vi "databasehandle.vi"(7 "condition":string, 8 "error in (no error)":errorcluster caption="错误输入（无错误）", 9 "columns":string[](array[string]), 10 "password":string="123", 11 "table":string) -> (0 "error out":errorcluster caption="错误输出", 3 "data":string[][](array[string]))   [LabVIEW 2016, in "潮位站数据传输.lvlib"]
uses:
  access/access.lvclass
  database_class/database.lvclass/database.ctl
  database_class/database.lvclass
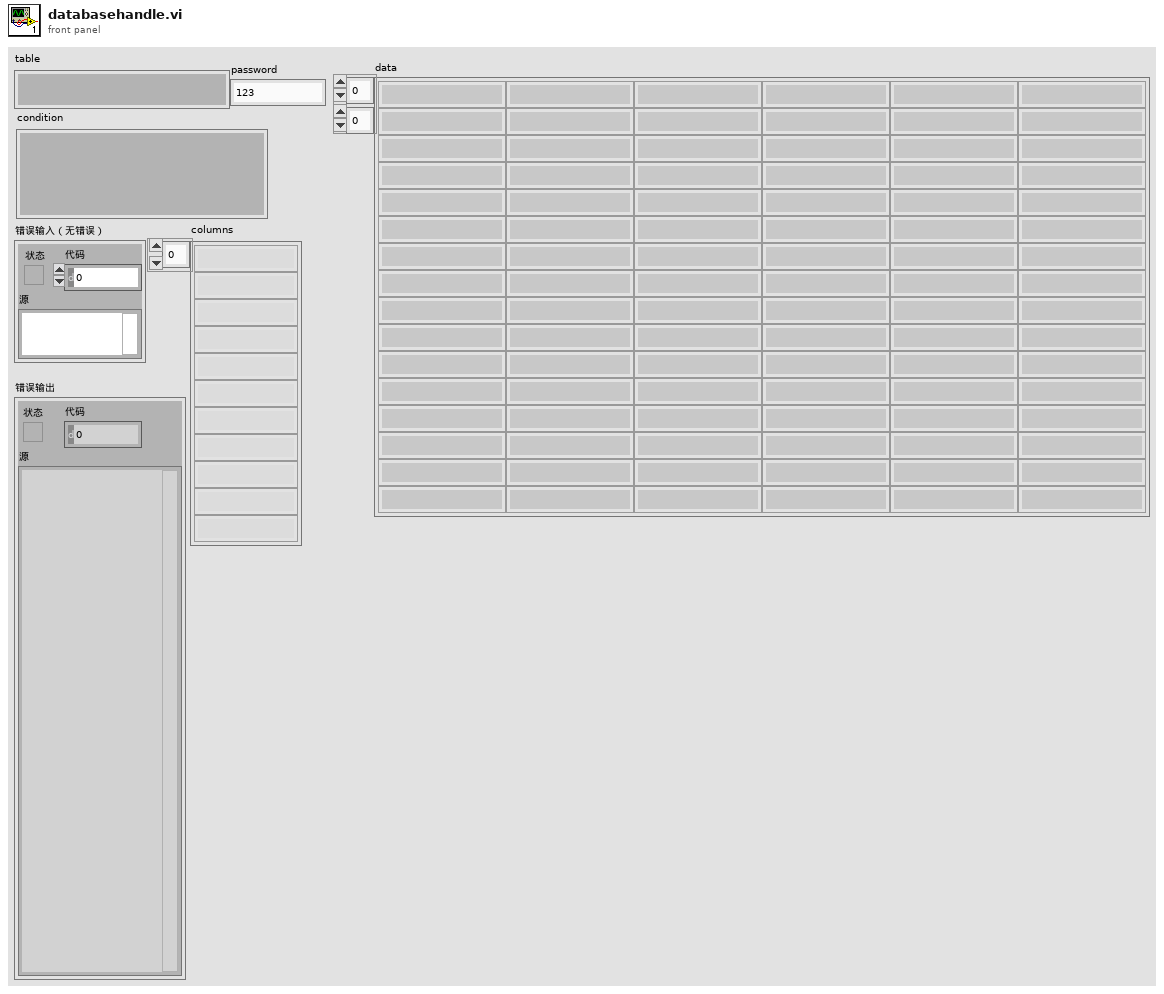
[diagram p1: front panel]
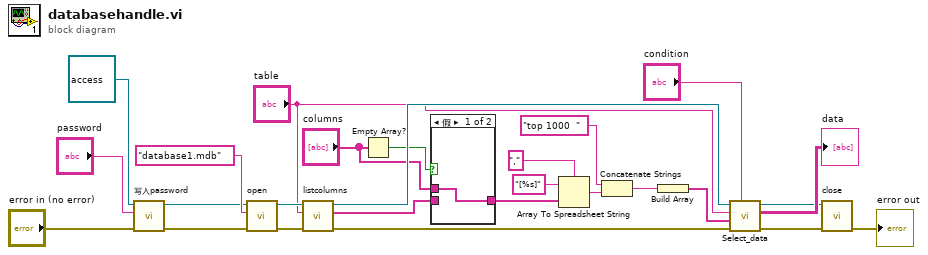
[diagram p0: block diagram]
diagram:
  n1 = call "写入password.vi"("error in (no error)"="error in (no error)", "password"="password", "database输入"=refnum<class "access.lvclass"> refnum ("access.lvclass")) -> ("error out"=w21:errorcluster, "database输出"=w23:refnum<class "access.lvclass">)  [unwired: 7 in]
  n2 = call-dynamic "open.vi"("error in (no error)"=w21, "database"="database1.mdb", "access 输入"=w23) -> ("error out"=w19:errorcluster, "access 输出"=w20:refnum<class "access.lvclass">)  [unwired: 7 in]
  n3 = call-dynamic "listcolumns.vi"("error in (no error)"=w19, "table"="table", "access 输入"=w20) -> ("error out"=w17:errorcluster, "columns"=w9:string[], "access 输出"=w18:refnum<class "access.lvclass">)  [unwired: 6 in]
  n4 = Empty Array?(array="columns") -> (empty?=w10:bool)
  n5 = case shown="假" w10 {
    tunnel: w9 -> [_ w28]
    tunnel: [w27 w28] -> w2
    tunnel: "columns" -> [w27 _]
    frame False {
    }
    frame True {
    }
  }
  n6 = Array To Spreadsheet String(delimiter (Tab)="," ("分隔符(Tab)"), array=w2, 3:"[%s]" ("格式字符串")) -> (spreadsheet string=w4:string)
  n7 = Concatenate Strings("top 1000  " ("字符串"), w4) -> (w3:string)
  n8 = Build Array(w3) -> (w1:string[])
  n9 = call-dynamic "Select_data.vi"("condition"="condition", "error in (no error)"=w17, "columns"=w1, "table"="table", "access 输入"=w18) -> ("error out"=w12:errorcluster, "data"=→"data":string[][], "access 输出"=w13:refnum<class "access.lvclass">)  [unwired: 4 in]
  n10 = call-dynamic "close.vi"("error in (no error)"=w12, "access 输入"=w13) -> ("error out"=→"error out":errorcluster)  [unwired: 8 in, 1 out]
